vi "Spectrum Measurements.vi"() -> ()   [LabVIEW 2011]
doc: "This Example shows results of the Spectrum Measurements Express VI. The Extract Portion of Signal Express VI is used to zoom into the most interesting area of the Result.\n\nThis example uses the following Express VIs: Simulate Signal, Spectal Measurements, Statistics, Formula, and Extract Portion of Signal."
uses:
  Instance           7 29Saved   Spectrum Measurements .vi
  Instance           1 29Saved   Spectrum Measurements .vi
  Instance           5 29Saved   Spectrum Measurements .vi
  Instance           6 29Saved   Spectrum Measurements .vi
  <vilib>/express/express analysis/Spectral/Block/exnSpectralBlock spectral measurements peak poly.vi
  <vilib>/express/express analysis/Spectral/Block/exnSpectralBlock spectral measurements peak DDT.vi
  <vilib>/express/express shared/transition.llb/Dynamic To Waveform Array.vi
  <vilib>/express/express shared/transition.llb/Waveform Array To Dynamic.vi
  <vilib>/express/express arith-compare/Formula/Block/exnFormulaBlock how many pts in the wave.vi
  <vilib>/express/express shared/ex_Modify Signal Name.vi
  <vilib>/express/express analysis/Spectral/XNode/ExpressSpectralMeasurementsBlockNode.xnode
  <vilib>/express/express arith-compare/Formula/XNode/ExpressFormulaBlockNode.xnode
panel:
  out "FFT Results (ZOOM)":dynamicdata(graph)=[{"t0"=timestamp(40 s since 1904-01-01), "dt"=10.0, "Y"=[0.0022259063596411074, 0.002288292026366782, 0.0023655874722497195, 0.002458551559375326, 0.002568202009910494, 0.0026958809381461744, 0.0028433382869280208, 0.003012840236132806, 0.003207313352573111, 0.0034305408091734467, 0.003687435713373986, 0.0039844307663187166, 0.004330047391056746, 0.004735749256962547, 0.005217261025030434, 0.005796677158775088, 0.00650597321639006, 0.007393141876255478, 0.008533566307432185, 0.010052708286100614, 0.012175849926609226, 0.015351853790435516, 0.020621813177117653, 0.031076102639714075, 0.061780541689127354, 1.99596920341715, 0.06715819594242894, 0.0333325894848088, 0.02229978387804661, 0.01682610147259099, 0.01355435135541218, 0.011377581276001388, 0.009824321273604714, 0.008659797917324371, 0.007753962212572111, 0.007028957151937819, 0.006435323708344039, 0.005940135979185554, 0.00552062610295718, 0.005160547714555612, 0.004847997193421876, 0.004574053626261719, 0.004331899721447642, 0.004116236298929308, 0.003922882009564225, 0.0037484933465449736, 0.0035903647878801946, 0.0034462835350003627, 0.003314422206300125, 0.003193258399820798], "attributes"=variant("SigName_"=variant(string "Sine"))}, {"t0"=timestamp(40 s since 1904-01-01), "dt"=10.0, "Y"=[3.158619370201504e-06, 3.7156822170270822e-06, 4.385059217869803e-06, 5.182394197563836e-06, 6.133240780103661e-06, 7.274462414481538e-06, 8.657188810367703e-06, 1.035178168094269e-05, 1.2455669714076319e-05, 1.5105598532695371e-05, 1.8497018311664447e-05, 2.2915471817212825e-05, 2.8788915591235352e-05, 3.6778024264739976e-05, 4.7938534265743104e-05, 6.402739710934487e-05, 8.811386971170397e-05, 0.00012588579877171853, 0.0001886883102719142, 0.00030139324002763265, 0.0005258815165854275, 0.001046479067549559, 0.002591711846986906, 0.010124662324760031, 0.9517417353587385, 1.998658373788234, 1.0484761890736607, 0.01139668780283256, 0.0027798251425649964, 0.0011012081819852424, 0.0005477126281063715, 0.00031196006893776946, 0.00019455742553211284, 0.00012951847547208923, 9.057683900272649e-05, 6.583537543109655e-05, 4.936153529314879e-05, 3.796766915252712e-05, 2.9835409023768585e-05, 2.3875293988050806e-05, 1.940722977396386e-05, 1.59916061939581e-05, 1.3335608084726551e-05, 1.1239041401188132e-05, 9.561863816774592e-06, 8.204103534651311e-06, 7.093091272757877e-06, 6.175139156344032e-06, 5.409997353008042e-06, 4.767086699652385e-06], "attributes"=variant("SigName_"=variant(string "Sine"))}, {"t0"=timestamp(40 s since 1904-01-01), "dt"=10.0, "Y"=[3.716070859869099e-06, 3.749869168719713e-06, 3.78813025023203e-06, 3.828676896986085e-06, 3.868566412061363e-06, 3.903839084744353e-06, 3.929170921622575e-06, 3.93740564487943e-06, 3.918951937871005e-06, 3.861087673679399e-06, 3.7474061448898934e-06, 3.5582978324762465e-06, 3.2756284764066427e-06, 2.9030656010720294e-06, 2.541663619330851e-06, 2.5722754357604084e-06, 3.5129087709805407e-06, 5.196921218680704e-06, 6.37701720882783e-06, 3.8383677747699036e-06, 1.9322159493006583e-05, 0.028758235332049364, 0.36649036736997337, 1.2551460295366257, 1.9235744145091471, 2.0000160419385757, 1.940930613929907, 1.3168006342868825, 0.4096058986024714, 0.036013277376535896, 2.5994277340837337e-05, 2.0595905576962163e-06, 4.1352507399613495e-06, 3.1394533710050713e-06, 2.0011637250809925e-06, 2.4397164032404638e-06, 3.4156258436863133e-06, 4.224030903753107e-06, 4.798327867000102e-06, 5.180172221068104e-06, 5.418406249240548e-06, 5.552758423048555e-06, 5.612922666516316e-06, 5.620488243804419e-06, 5.591014259068352e-06, 5.535698310417706e-06, 5.462612128381945e-06, 5.3775884985407005e-06, 5.284852095790849e-06, 5.187467051549578e-06], "attributes"=variant("SigName_"=variant(string "Sine"))}]
  out "FFT Results (Lin)":dynamicdata(graph)=[{"t0"=timestamp(0 s since 1904-01-01), "dt"=10.0, "Y"=array[500 elements], "attributes"=variant("SigName_"=variant(string "Sine"))}, {"t0"=timestamp(0 s since 1904-01-01), "dt"=10.0, "Y"=array[500 elements], "attributes"=variant("SigName_"=variant(string "Sine"))}, {"t0"=timestamp(0 s since 1904-01-01), "dt"=10.0, "Y"=array[500 elements], "attributes"=variant("SigName_"=variant(string "Sine"))}]
  out "FFT Results (Log)":dynamicdata(graph)=[{"t0"=timestamp(0 s since 1904-01-01), "dt"=10.0, "Y"=array[500 elements], "attributes"=variant("SigName_"=variant(string "Sine"))}, {"t0"=timestamp(0 s since 1904-01-01), "dt"=10.0, "Y"=array[500 elements], "attributes"=variant("SigName_"=variant(string "Sine"))}, {"t0"=timestamp(0 s since 1904-01-01), "dt"=10.0, "Y"=array[500 elements], "attributes"=variant("SigName_"=variant(string "Sine"))}]
  in  "Frequency":dbl(slide)=290.3225806451613 scale=0.0..5000.0
  out "Signal":dynamicdata(graph)=[{"t0"=timestamp(3087498156.8319855 s since 1904-01-01), "dt"=0.0001, "Y"=array[1000 elements], "attributes"=variant("SigName_"=variant(string "Sine"))}]
  in  "stop":bool
  # "This Example shows results of the Spectrum Measurements Express VI.\nThe Extract Portion of Signal Express VI is used to zoom into the most interesting area of the Result."
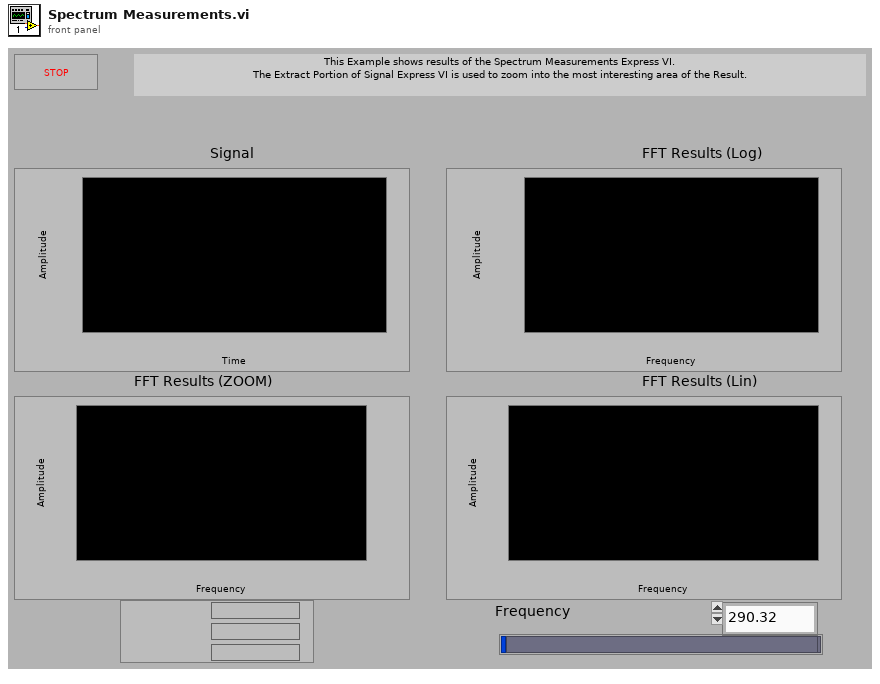
[diagram p1: front panel]
types:
  T1 = cluster{"averaging mode":u16, "weighting mode":u16, "number of averages":u32}
  T2 = cluster{"dB On (F)":bool, "unwrap phase (F)":bool, "convert to degree (F)":bool}
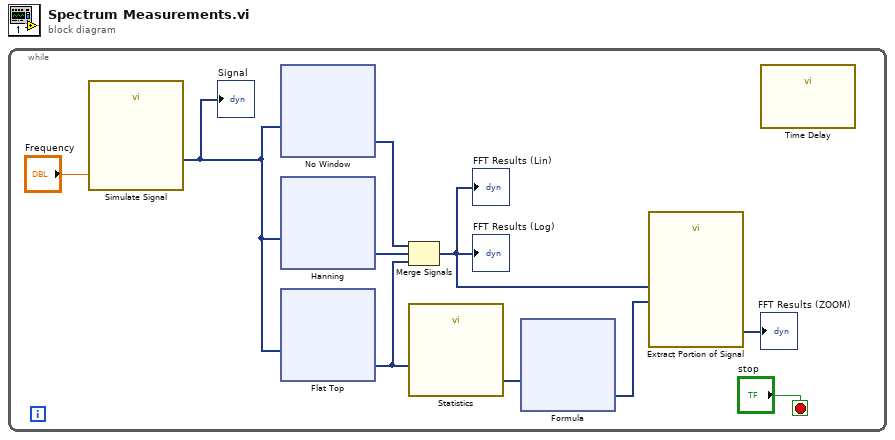
[diagram p0: block diagram]
diagram:
  n1 = while {
    stop <- "stop" stop-if-true
    n2 = call "Simulate Signal"("Frequency"="Frequency") -> ("Sine"=w6:dynamicdata)  [unwired: 13 in, 1 out]
    "Signal" <- w6
    n3 = xnode "No Window"("Signals"=w6) -> ("FFT - (Peak)"=w8:dynamicdata)  [unwired: 1 in, 2 out]
    n4 = xnode "Hanning"("Signals"=w6) -> ("FFT - (Peak)"=w7:dynamicdata)  [unwired: 1 in, 2 out]
    n5 = xnode "Flat Top"("Signals"=w6) -> ("FFT - (Peak)"=w5:dynamicdata)  [unwired: 1 in, 2 out]
    n6 = Merge Signals(w8, w7, w5) -> (w3:dynamicdata)
    "FFT Results (Log)" <- w3
    "FFT Results (Lin)" <- w3
    n7 = call "Statistics"("Signals"=w5) -> ("Index of Max"=w4:dynamicdata)  [unwired: 25 in, 1 out]
    n8 = xnode "Formula"("MaxIndex"=w4) -> ("Result"=w2:dynamicdata)  [unwired: 1 in, 1 out]
    n9 = call "Extract Portion of Signal"("Begin Sample"=w2, "Signals"=w3) -> ("Section"=→"FFT Results (ZOOM)":dynamicdata)  [unwired: 8 in, 1 out]
    n10 = call "Time Delay"() -> ()  [unwired: 11 in, 1 out]
  }
